vi "initialise Channel.vi"(8 "error in (no error)":errorcluster, 10 "channel":u32, 11 "pumpIndex":u32) -> (0 "error out":errorcluster, 3 "function return":i32)   [LabVIEW 2018]
doc: "extern ASIAPUMP_INTERFACE_API BOOL initialiseChannel( unsigned int pumpIndex ,\n unsigned int channel );"
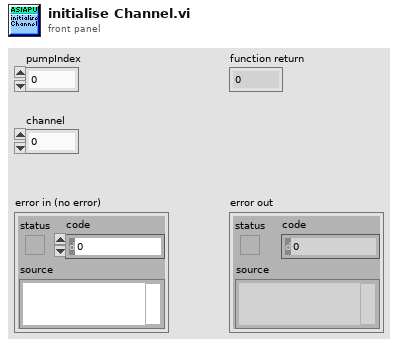
[diagram p1: front panel]
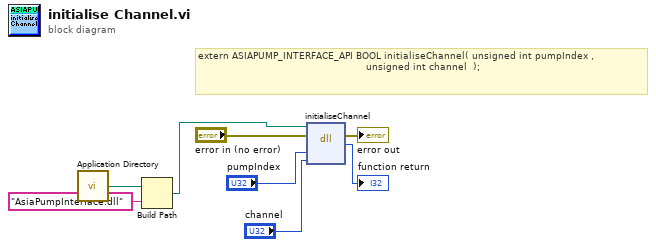
[diagram p0: block diagram]
diagram:
  # "extern ASIAPUMP_INTERFACE_API BOOL initialiseChannel( unsigned int pumpIndex ,\n                                                        unsigned int channel  );"
  n1 = call <vilib>:"Application Directory.vi"() -> ("Application Directory"=w3:path)
  n2 = Build Path(base path=w3, name or relative path="AsiaPumpInterface.dll") -> (appended path=w1:path)
  n3 = dll-call lib="C:/Program Files (x86)/National Instruments/LabVIEW 2018/user.lib/AsiaPumpInterface/AsiaPumpInterface.*" fn="initialiseChannel"(path in=w1, error in="error in (no error)", "pumpIndex"="pumpIndex", "channel"="channel") -> (error out=→"error out":errorcluster, "return type"=→"function return":i32)  [unwired: 3 in, 1 out]
